vi "Stereo Logitech Loop.vi"() -> ()   [LabVIEW 2012]
uses:
  <vilib>/Platform/TimedLoop/XDataNode/timing_clust.ctl
  <vilib>/Platform/TimedLoop/XDataNode/nitl_modes.ctl
  <vilib>/Platform/TimedLoop/XDataNode/wakeup.ctl
  <vilib>/Platform/TimedLoop/XDataNode/XDataNode.xnode
  <vilib>/Platform/TimedLoop/XDataNode/XDNodeRunTimeDep.lvlib
  <vilib>/vision/NI_Vision_Development_Module.lvlib
panel:
  in  "Debug":bool
  in  "stop?":bool caption="Stop (F)"
  out "Gauge":cluster{dbl, dbl}(knob) scale=0.0..50.0
  in  "Left Image":path
  in  "Right Image":path
  out "XY Graph 2":cluster{dbl[], dbl[]}(graph)
  out "XY Graph":cluster{dbl[], dbl[]}(graph)
  out "Right Image":T1(plugin-control)
  out "Left Image":T1(plugin-control)
  in  "Record Button":bool
  in  "Save File Path":path
  out "Time Stamp":timestamp
  out "Image Index":dbl
  out "error out":errorcluster
  in  "error in":errorcluster
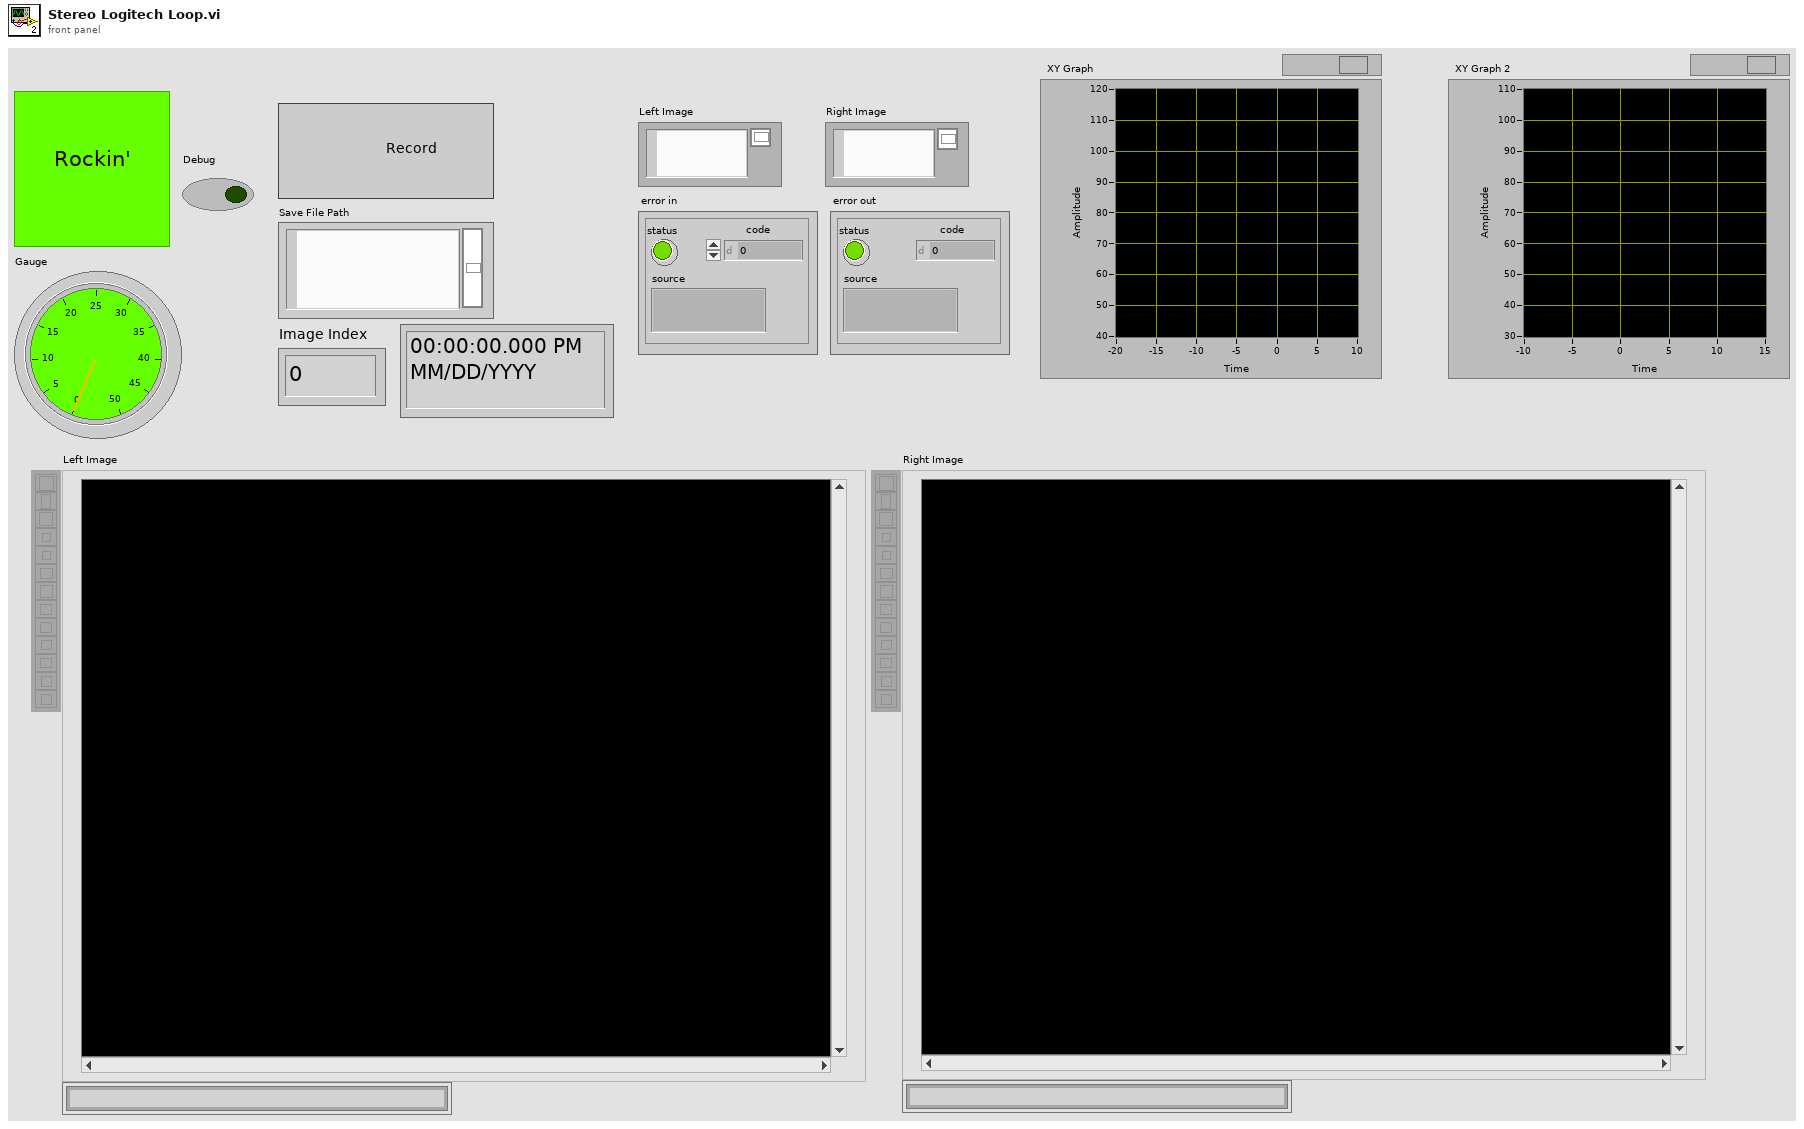
[diagram p1: front panel]
types:
  T1 = typedef "IMAQ Image.ctl" = refnum<image>
  T2 = typedef "Image Type" = u32
  T3 = typedef "XDNodeRunTimeDep.lvlib/timing_clust.ctl" = cluster{"Expected End [f-1]":u64, "Actual End [f-1]":u64, "Finished Late? [f-1]":bool, "Expected End [i-1]":u64, "Actual End [i-1]":u64, "Finished Late? [i-1]":bool, "Expected Start [i]":u64, "Actual Start [i]":u64, "Expected Start [f]":u64, "Actual Start [f]":u64, "Source Name":string, "Structure Name":string, "Period":i64, "Deadline":i64, "Offset":i64, "Start":i64, "Priority":i32, "Timeout":i32, "Mode":T4, "Wakeup Reason":T5, "Error":errorcluster, "Source Type":string, "Secondary Source Type":string, "Global End Time":u64, "Global Start Time":u64, "Frame Duration":u64, "Iteration Duration":u64, "Assigned CPU":i32, "I/O Scan Engine Mode":u32}
  T4 = typedef "XDNodeRunTimeDep.lvlib/nitl_modes.ctl" = enum32{"No Change", "Process missed periods, maintain original phase", "Discard missed periods, maintain original phase", "Process missed periods, ignore original phase", "Discard missed periods, ignore original phase"}
  T5 = typedef "XDNodeRunTimeDep.lvlib/wakeup.ctl" = enum32{"Normal", "Aborted", "Asynchronous wakeup", "Timing source error", "Timed loop error", "Timeout"}
  T6 = cluster{"Start Point":cluster{"X":sgl, "Y":sgl}, "End Point":cluster{"X":sgl, "Y":sgl}, "Length":dbl, "Orientation":dbl, "Score":dbl}[]
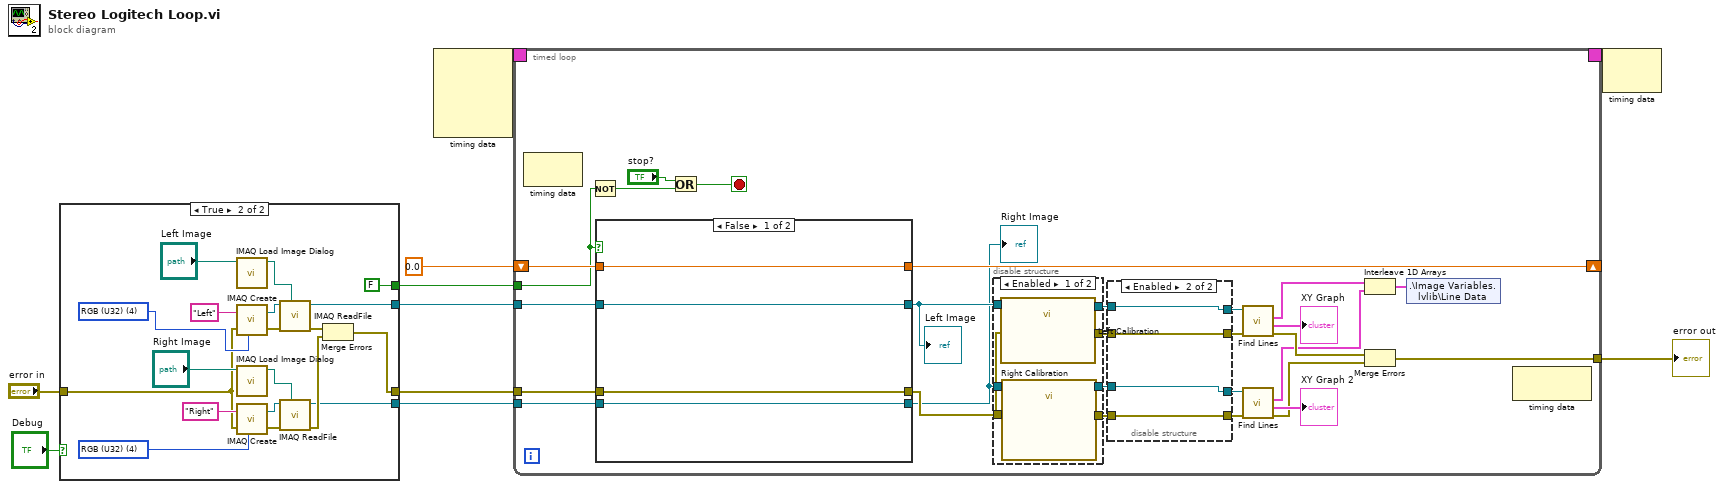
[diagram p0: block diagram]
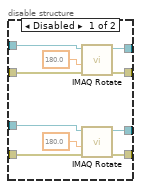
[diagram p3: hidden frame]
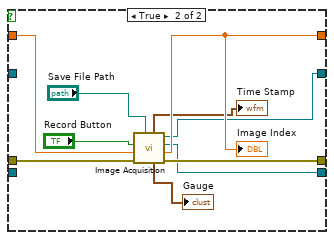
[diagram p4: hidden frame]
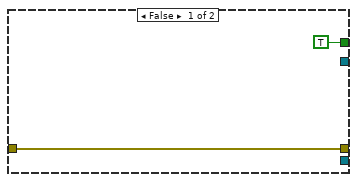
[diagram p5: hidden frame]
diagram:
  n1 = case shown="True" "Debug" {
    tunnel: "error in" -> [w11 w17]
    tunnel: [w11 w16] -> w6
    tunnel: [TRUE FALSE] -> w5
    tunnel: [_ w14] -> w4
    tunnel: [_ w13] -> w3
    frame False {
    }
    frame True {
      w24 = T2 4 items=["Grayscale (U8)", "Grayscale (I16)", "Grayscale (SGL)", "Complex (CSG)", "RGB (U32)", "HSL (U32)", "RGB (U64)", "Grayscale (U16)"] ("Image Type")
      w29 = T2 4 items=["Grayscale (U8)", "Grayscale (I16)", "Grayscale (SGL)", "Complex (CSG)", "RGB (U32)", "HSL (U32)", "RGB (U64)", "Grayscale (U16)"] ("Image Type")
      n2 = call "IMAQ Load Image Dialog"("Start Path"="Left Image") -> ("Path"=w30:path)  [unwired: 8 in, 2 out]
      n3 = call "IMAQ Create"("Image Name"="Left", "Image Type"=w24, "error in (no error)"=w17) -> ("New Image"=w25:T1, "error out"=w26:errorcluster)  [unwired: 2 in]
      n4 = call "IMAQ Load Image Dialog"("Start Path"="Right Image") -> ("Path"=w31:path)  [unwired: 8 in, 2 out]
      n5 = call "IMAQ Create"("Image Name"="Right", "Image Type"=w29, "error in (no error)"=w17) -> ("New Image"=w28:T1, "error out"=w27:errorcluster)  [unwired: 2 in]
      n6 = call "IMAQ ReadFile"("File Path"=w30, "error in (no error)"=w26, "Image"=w25) -> ("error out"=w22:errorcluster, "Image Out"=w13:T1)  [unwired: 4 in, 3 out]
      n7 = call "IMAQ ReadFile"("File Path"=w31, "error in (no error)"=w27, "Image"=w28) -> ("error out"=w23:errorcluster, "Image Out"=w14:T1)  [unwired: 4 in, 3 out]
      n8 = Merge Errors(w22, w23) -> (w16:errorcluster)
    }
  }
  n9 = node-c288() -> (w2:T3)  [unwired: 4 in]
  n10 = timed-loop {
    tunnel: w6 -> [w59]
    shift-right: [w57] -> _
    shift-left: 0.0 ("Image Index In") -> [w58]
    tunnel: [w56] -> w9
    tunnel: w5 -> [w53]
    tunnel: w4 -> [w55]
    tunnel: w3 -> [w54]
    timing: w2 -> [_]
    timing-out: [_] -> w1
    stop <- w52 stop-if-true
    n11 = node-c288() -> ()  [unwired: 1 in, 1 out]
    n12 = Not(x=w53) -> (.not. x?=w51:bool)
    n13 = case shown="False" w53 {
      tunnel: w59 -> [w86 w97]
      tunnel: w58 -> [w87 w96]
      tunnel: [w86 w95] -> w50
      tunnel: [w87 w94] -> w57
      tunnel: [w84 w93] -> w45
      tunnel: [w85 w92] -> w44
      tunnel: w55 -> [w85 _]
      tunnel: w54 -> [w84 _]
      frame False {
      }
      frame True {
        n14 = call "Image Acquisition.vi"("Save File Path"="Save File Path", "Error In"=w97, "Image Index In"=w96, "Record Button"="Record Button") -> ("Error Out"=w95:errorcluster, "Image Index Out"=w94:dbl, "Right Image"=w92:T1, "Left Image"=w93:T1, "Gauge"=→"Gauge":cluster{dbl, dbl}, "Time Stamp"=→"Time Stamp":timestamp)  [unwired: 2 in]
        "Image Index" <- w94
      }
    }
    "Left Image" <- w45
    "Right Image" <- w44
    n15 = Or(x="stop?", y=w51) -> (x .or. y?=w52:bool)
    n16 = disable-structure shown="Enabled" {
      disable-tunnel: w50 -> [w66 w67]
      disable-tunnel: w45 -> [w65 w69]
      disable-tunnel: w44 -> [w64 w68]
      disable-tunnel: [w63 w69] -> w41
      disable-tunnel: [w62 w67] -> w38
      disable-tunnel: [w61 w68] -> w37
      disable-tunnel: [w60 w67] -> w34
      frame Enabled {
        n17 = call "Left Calibration"("Image In"=w65, "error in"=w66) -> ("Image Out"=w63:T1, "error out"=w62:errorcluster)  [unwired: 24 in]
        n18 = call "Right Calibration"("Image In"=w64, "error in"=w66) -> ("Image Out"=w61:T1, "error out"=w60:errorcluster)  [unwired: 24 in]
      }
      frame Disabled {
      }
    }
    n19 = disable-structure shown="Enabled" {
      disable-tunnel: w41 -> [w77 w83]
      disable-tunnel: [w76 w83] -> w40
      disable-tunnel: [w75 w82] -> w39
      disable-tunnel: w38 -> [w74 w82]
      disable-tunnel: w37 -> [w73 w81]
      disable-tunnel: [w72 w81] -> w36
      disable-tunnel: [w71 w80] -> w35
      disable-tunnel: w34 -> [w70 w80]
      frame Disabled {
        n20 = call "IMAQ Rotate"("error in (no error)"=w74, "Angle (degrees)"=sgl 180.0, "Image Src"=w77) -> ("error out"=w75:errorcluster, "Image Dst Out"=w76:T1)  [unwired: 7 in]
        n21 = call "IMAQ Rotate"("error in (no error)"=w70, "Angle (degrees)"=sgl 180.0, "Image Src"=w73) -> ("error out"=w71:errorcluster, "Image Dst Out"=w72:T1)  [unwired: 7 in]
      }
      frame Enabled {
      }
    }
    n22 = call "Find Lines.vi"("error in"=w39, "Image In"=w40) -> ("error out"=w48:errorcluster, "XY Graph"=→"XY Graph":cluster{dbl[], dbl[]}, "Lines Calibrated (Shape Detection 1)"=w43:T6)  [unwired: 6 in, 1 out]
    n23 = call "Find Lines.vi"("error in"=w35, "Image In"=w36) -> ("error out"=w46:errorcluster, "XY Graph"=→"XY Graph 2":cluster{dbl[], dbl[]}, "Lines Calibrated (Shape Detection 1)"=w42:T6)  [unwired: 6 in, 1 out]
    n24 = Interleave 1D Arrays(w43, w42) -> (w33:T6)
    n25 = Merge Errors(w48, w46) -> (w56:errorcluster)
    n26 = shared-variable ".\\Image Variables.lvlib\\Line Data"(w33) -> ()  [unwired: 1 in, 1 out]
    n27 = node-c288() -> ()  [unwired: 1 in, 1 out]
  }
  "error out" <- w9
  n28 = node-c288(w1) -> ()  [unwired: 1 out]
